vi "Keithley2200series_Start2.vi"(0 "VISA In":refnum<visa-resource-name>, 1 "Function(0:Voltage) 3":u16(ring) items=["Voltage", "Current"], 2 "Out set":dbl, 3 "Err In":errorcluster, 4 "Cml set":dbl) -> (5 "VISA out":refnum<visa-resource-name>, 6 "Meas Func":i32, 7 "Err Out":errorcluster)   [LabVIEW 2014]
uses:
  C:/Users/rad/Desktop/Keithley 2200 Series Power Supplies Ver 1.2 (LV2009)/Keithley 2200 Series/Keithley 2200 Series.lvlib
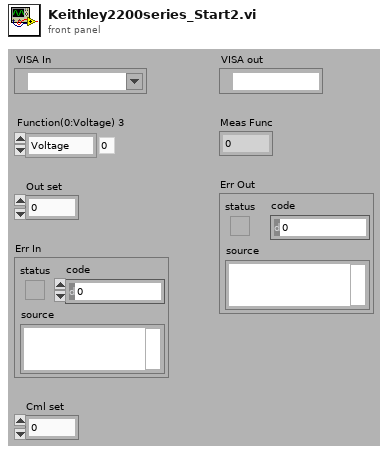
[diagram p1: front panel]
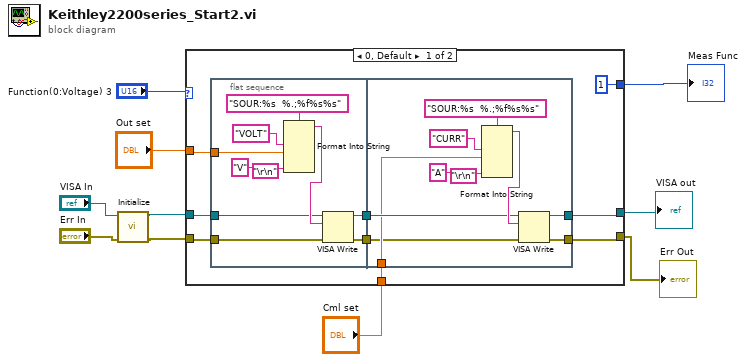
[diagram p0: block diagram]
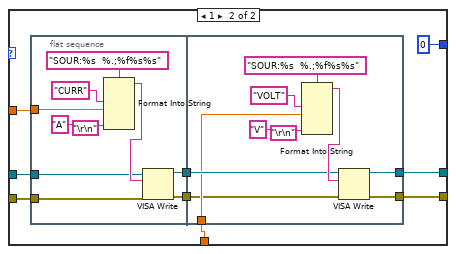
[diagram p2: hidden frame]
diagram:
  n1 = call "Initialize.vi"("error in (no error)"="Err In", "VISA resource name"="VISA In") -> ("error out"=w1:errorcluster, "VISA resource name out"=w2:refnum<visa-resource-name>)  [unwired: 8 in]
  n2 = case shown="0, Default" "Function(0:Voltage) 3" {
    tunnel: "Out set" -> [w19 w46]
    tunnel: "Cml set" -> [w17 w45]
    tunnel: w2 -> [w12 w44]
    tunnel: w1 -> [w11 w43]
    tunnel: [w15 w42] -> w6
    tunnel: [w14 w41] -> w5
    tunnel: [1 0] -> w10
    frame 0, Default {
      n3 = flat-sequence {
        tunnel: w19 -> [w27]
        tunnel: [w23] -> w18
        tunnel: [w22] -> w16
        tunnel: w12 -> [w21]
        tunnel: w11 -> [w20]
        tunnel: w18 -> [w34]
        tunnel: w17 -> [w33]
        tunnel: w16 -> [w32]
        tunnel: [w31] -> w15
        tunnel: [w30] -> w14
        frame #0 {
          n4 = Format Into String(format string="SOUR:%s  %.;%f%s%s", "VOLT" ("format string"), w27, "V" ("input 3"), "\r\n" ("End of Line Constant")) -> (resulting string=w24:string)  [unwired: 2 in, 1 out]
          n5 = VISA Write(VISA resource name=w21, write buffer=w24, error in (no error)=w20) -> (VISA resource name out=w23:refnum<visa-resource-name>, error out=w22:errorcluster)  [unwired: 1 out]
        }
        frame #1 {
          n6 = Format Into String(format string="SOUR:%s  %.;%f%s%s", "CURR" ("format string"), w33, "A" ("input 3"), "\r\n" ("End of Line Constant")) -> (resulting string=w35:string)  [unwired: 2 in, 1 out]
          n7 = VISA Write(VISA resource name=w34, write buffer=w35, error in (no error)=w32) -> (VISA resource name out=w31:refnum<visa-resource-name>, error out=w30:errorcluster)  [unwired: 1 out]
        }
      }
    }
    frame 1 {
      n8 = flat-sequence {
        tunnel: w46 -> [w56]
        tunnel: [w52] -> w48
        tunnel: [w51] -> w47
        tunnel: w44 -> [w50]
        tunnel: w43 -> [w49]
        tunnel: w48 -> [w63]
        tunnel: w45 -> [w62]
        tunnel: w47 -> [w61]
        tunnel: [w60] -> w42
        tunnel: [w59] -> w41
        frame #0 {
          n9 = Format Into String(format string="SOUR:%s  %.;%f%s%s", "CURR" ("format string"), w56, "A" ("input 3"), "\r\n" ("End of Line Constant")) -> (resulting string=w53:string)  [unwired: 2 in, 1 out]
          n10 = VISA Write(VISA resource name=w50, write buffer=w53, error in (no error)=w49) -> (VISA resource name out=w52:refnum<visa-resource-name>, error out=w51:errorcluster)  [unwired: 1 out]
        }
        frame #1 {
          n11 = Format Into String(format string="SOUR:%s  %.;%f%s%s", "VOLT" ("format string"), w62, "V" ("input 3"), "\r\n" ("End of Line Constant")) -> (resulting string=w64:string)  [unwired: 2 in, 1 out]
          n12 = VISA Write(VISA resource name=w63, write buffer=w64, error in (no error)=w61) -> (VISA resource name out=w60:refnum<visa-resource-name>, error out=w59:errorcluster)  [unwired: 1 out]
        }
      }
    }
  }
  "VISA out" <- w6
  "Err Out" <- w5
  "Meas Func" <- w10
